vi "LCR_Readout.vi"(8 "error in (no error)":errorcluster, 9 "CurrentVolts":dbl, 10 "Frequency in Hz":i32, 11 "WK6440B in":refnum<class "WK6440B.lvclass">) -> (0 "error out":errorcluster, 1 "Resistance in Ohm":dbl, 2 "Capacitance in pF":dbl, 3 "WK6440B out":refnum<class "WK6440B.lvclass">)   [LabVIEW 2018, in "WK6440B.lvclass"]
uses:
  WK6440B.lvclass
  C:/ProbeTestSoftware2019/itk-strip-sensor-qc/InstrControl/InstrControl.lvclass
  InstrControl.lvclass
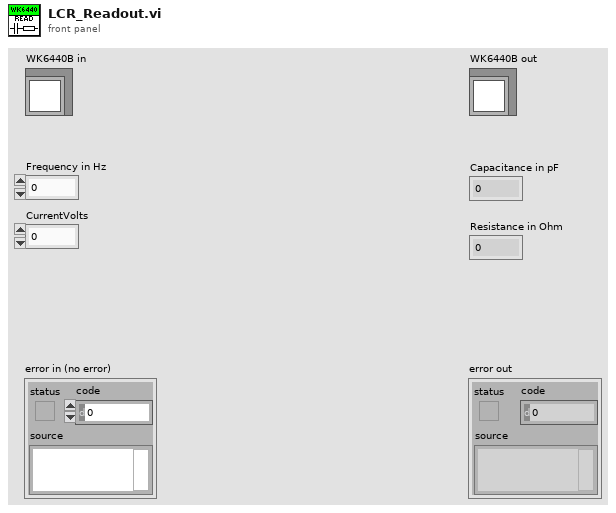
[diagram p1: front panel]
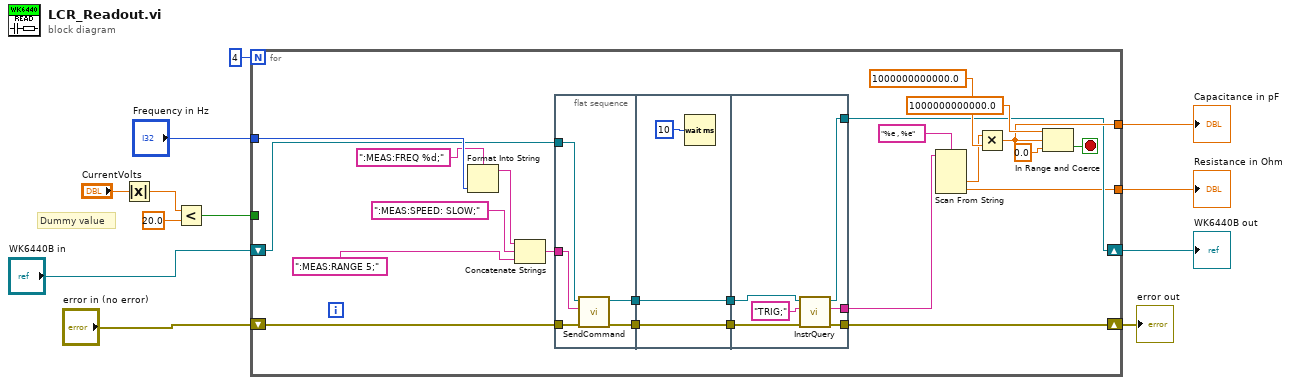
[diagram p0: block diagram]
diagram:
  # "Dummy value"
  n1 = Absolute Value(x="CurrentVolts") -> (abs(x)=w3:dbl)
  n2 = Less?(x=w3, y=20.0) -> (x < y?=w1:bool)
  n3 = for {
    N: 4 -> [_]
    tunnel: [w14] -> w8
    tunnel: [w32] -> w9
    tunnel: "Frequency in Hz" -> [w30]
    shift-right: [w15] -> w5
    shift-left: "WK6440B in" -> [w22]
    shift-right: [w20] -> w10
    shift-left: "error in (no error)" -> [w29]
    tunnel: w1 -> [_]
    stop <- w31 stop-if-true
    n4 = Format Into String(format string=":MEAS:FREQ %d;", w30) -> (resulting string=w28:string)  [unwired: 2 in, 1 out]
    n5 = Concatenate Strings(w28, ":MEAS:SPEED: SLOW;", ":MEAS:RANGE 5;") -> (w35:string)
    n6 = flat-sequence {
      tunnel: w35 -> [w38]
      tunnel: w29 -> [w40]
      tunnel: w22 -> [w36]
      tunnel: [w39] -> w19
      tunnel: [w37] -> w17
      tunnel: w19 -> [w42]
      tunnel: [w42] -> w18
      tunnel: w17 -> [w41]
      tunnel: [w41] -> w16
      tunnel: [w48] -> w20
      tunnel: [w47] -> w21
      tunnel: w18 -> [w49]
      tunnel: w16 -> [w45]
      tunnel: [w44] -> w15
      frame #0 {
        n7 = call "SendCommand.vi"("error in (no error)"=w40, "Command string"=w38, "InstControl in"=w36) -> ("error out"=w39:errorcluster, "InstControl out"=w37:refnum<class "WK6440B.lvclass">)  [unwired: 7 in]
      }
      frame #1 {
        n8 = Wait (ms)(milliseconds to wait=10) -> ()  [unwired: 1 out]
      }
      frame #2 {
        n9 = call-dynamic "InstrQuery.vi"("error in (no error)"=w49, "Command string"="TRIG;", "InstControl in"=w45) -> ("error out"=w48:errorcluster, "Instrument response"=w47:string, "InstControl out"=w44:refnum<class "WK6440B.lvclass">)  [unwired: 6 in]
      }
    }
    n10 = Scan From String(format string="%e , %e", input string=w21) -> (output 1=w23:dbl, output 2=w14:dbl)  [unwired: 4 in, 3 out]
    n11 = Multiply(x=w23, y=1000000000000.0) -> (x*y=w32:dbl)
    n12 = In Range and Coerce(upper limit=1000000000000.0 ("y"), x=w32, lower limit=0.0) -> (In Range?=w31:bool)  [unwired: 1 out]
  }
  "error out" <- w10
  "WK6440B out" <- w5
  "Capacitance in pF" <- w9
  "Resistance in Ohm" <- w8
